vi "MagX Find Experiment.vi"(8 "error in":errorcluster, 9 "Time Stamp":timestamp, 10 "Location":string, 11 "Data in":T1[](array[typedef])) -> (0 "error out":errorcluster, 3 "Data out":T1[](array[typedef]))   [LabVIEW 2024]
uses:
  Experiment info.ctl
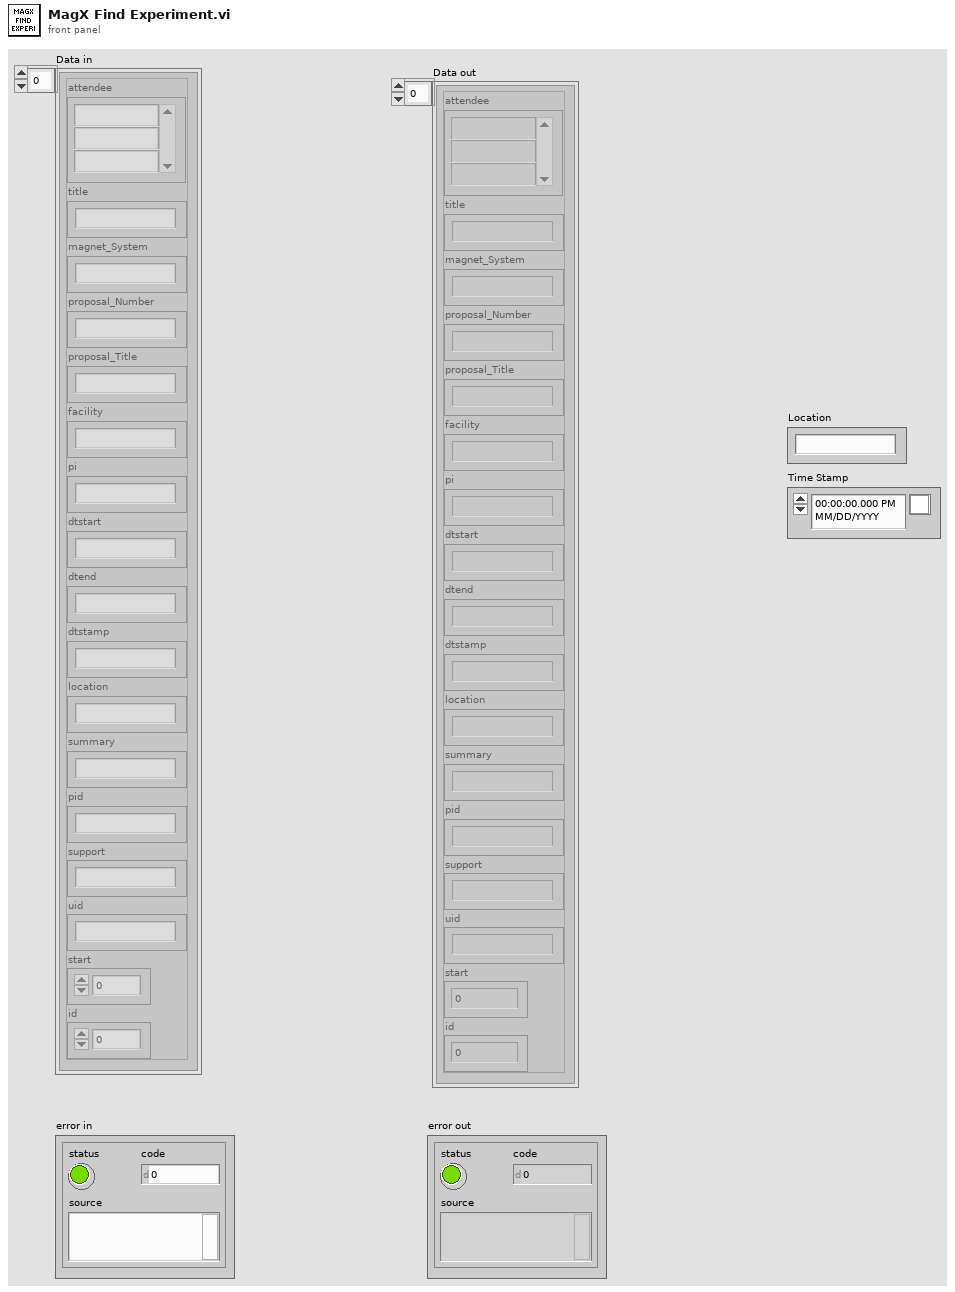
[diagram p1: front panel]
types:
  T1 = typedef "Experiment info.ctl" = cluster{"attendee":string[], "title":string, "magnet_System":string, "proposal_Number":string, "proposal_Title":string, "facility":string, "pi":string, "dtstart":string, "dtend":string, "dtstamp":string, "location":string, "summary":string, "pid":string, "support":string, "uid":string, "start":u64, "id":u64}
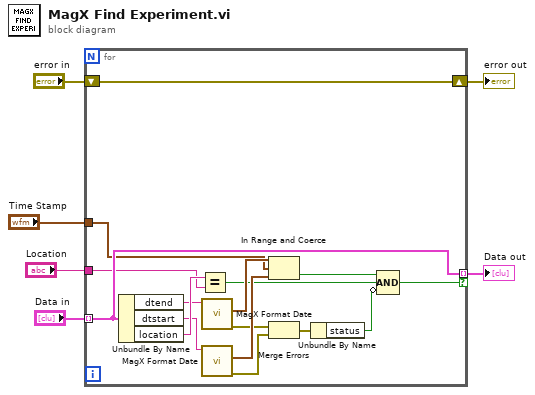
[diagram p0: block diagram]
diagram:
  n1 = for {
    tunnel: "Data in" -> [w22] mode=indexing
    tunnel: [w22] -> w5 mode=indexing if=w13
    tunnel: "Location" -> [w20]
    tunnel: "Time Stamp" -> [w15]
    shift-right: [w12] -> w1
    shift-left: "error in" -> [w12]
    n2 = Unbundle By Name(w22) -> ("dtend"=w19:string, "dtstart"=w18:string, "location"=w21:string)
    n3 = Equal?(x=w21, y=w20) -> (x = y?=w7:bool)
    n4 = call "MagX Format Date.vi"("String"=w19) -> ("error out"=w11:errorcluster, "Timestamp"=w17:timestamp)  [unwired: 8 in, 1 out]
    n5 = call "MagX Format Date.vi"("String"=w18) -> ("error out"=w10:errorcluster, "Timestamp"=w16:timestamp)  [unwired: 8 in, 1 out]
    n6 = In Range and Coerce(upper limit=w17, x=w15, lower limit=w16) -> (In Range?=w14:bool)  [unwired: 1 out]
    n7 = Merge Errors(w11, w10) -> (w9:errorcluster)
    n8 = Unbundle By Name(w9) -> ("status"=w8:bool)
    n9 = Compound Arithmetic op=AND(w14, w7, invert w8) -> (w13:bool)
  }
  "Data out" <- w5
  "error out" <- w1
